vi "Configure Modulation Low Level (Deviation).vi"(8 "error in (no error)":errorcluster, 9 "Deviation":dbl=1.0, 10 "Modulation (FM)":enum16{"FM", "PM", "PWM"}(ring), 11 "VISA resource name":refnum<visa-resource-name>) -> (0 "error out":errorcluster, 3 "VISA resource name out":refnum<visa-resource-name>)   [LabVIEW 2017, in "Keithley 3390.lvlib"]
uses:
  Keithley 3390.lvlib
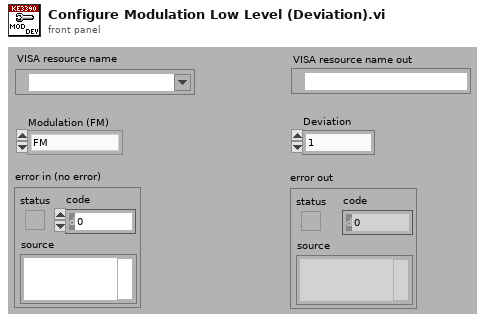
[diagram p1: front panel]
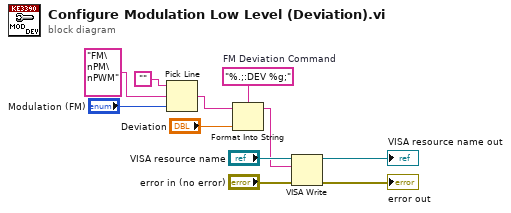
[diagram p0: block diagram]
diagram:
  w8 = "%.;:DEV %g;"  # FM Deviation Command
  n1 = Pick Line(string ("")="", multi-line string="FM\nPM\nPWM", line index="Modulation (FM)") -> (output string=w4:string)
  n2 = Format Into String(format string=w8, initial string=w4, "Deviation") -> (resulting string=w10:string)  [unwired: 1 in, 1 out]
  n3 = VISA Write(VISA resource name="VISA resource name", write buffer=w10, error in (no error)="error in (no error)") -> (VISA resource name out=→"VISA resource name out":refnum<visa-resource-name>, error out=→"error out":errorcluster)  [unwired: 1 out]
